vi "1820 PS Heat duration.vi"(10 "PS Heat":bool, 11 "time stamp":timestamp format="%<%I:%M:%S %p>T") -> (3 "PS Heat on (HH:MM:SS)":dbl format="%<%H:%M:%S>t")   [LabVIEW 2019, in "Instrument.Oxford1820.lvclass"]
uses:
  Instrument.Oxford1820.lvclass
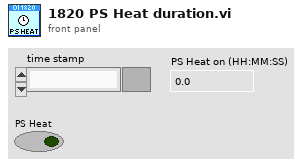
[diagram p1: front panel]
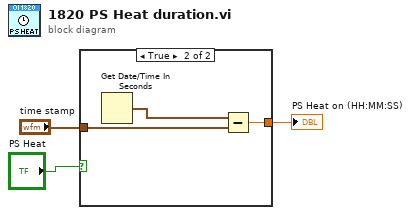
[diagram p0: block diagram]
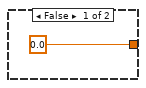
[diagram p2: hidden frame]
diagram:
  n1 = case shown="True" "PS Heat" {
    tunnel: "time stamp" -> [_ w7]
    tunnel: [0.0 w6] -> w2
    frame False {
    }
    frame True {
      n2 = Get Date/Time In Seconds() -> (seconds since 1Jan1904=w5:timestamp)
      n3 = Subtract(x=w5, y=w7) -> (x-y=w6:dbl)
    }
  }
  "PS Heat on (HH:MM:SS)" <- w2
